vi "VALVE & PUMP.vi"() -> ()   [LabVIEW 2011]
panel:
  out "trans_pump":bool
  out "ingr1_valve":bool
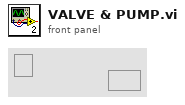
[diagram p1: front panel]
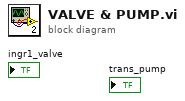
[diagram p0: block diagram]
diagram:
